vi "P4CMDSub Get Changelist Info.vi"(6 "operation message":string, 8 "error in (no error)":errorcluster, 9 "files":path[](array[path]), 10 "changelist":string, 11 "source control reference in":T1) -> (0 "error out":errorcluster, 1 "description":string, 2 "status":string, 3 "source control reference out":T1, 4 "changelist files array":string[](array[string]), 5 "date":string)   [LabVIEW 2020, in "NI_SCC_P4CMD.lvlib"]
uses:
  <vilib>/SourceControl/Providers/P4CMD/NI_SCC_P4CMD.lvlib
  <vilib>/SourceControl/sccapi/SCCAPI Refnum.ctl
  <vilib>/SourceControl/Providers/P4CMD/P4CMD Operations.ctl
  <vilib>/SourceControl/sccapi/NI_SCC.lvlib
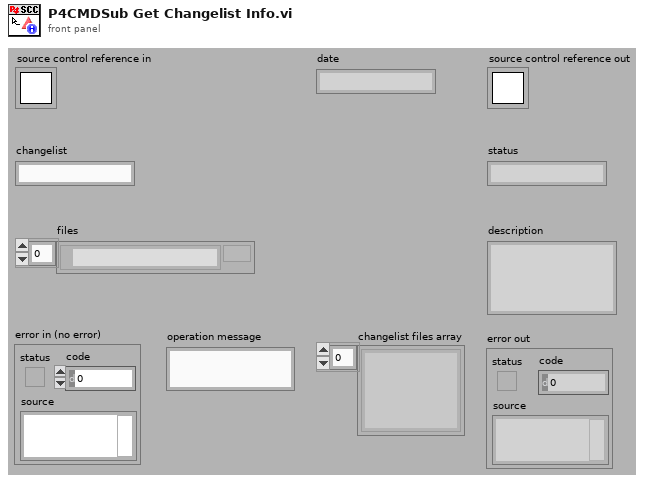
[diagram p1: front panel]
types:
  T1 = typedef "NI_SCC.lvlib/SCCAPI Refnum.ctl" = refnum<k1>
  T2 = typedef "NI_SCC_P4CMD.lvlib/P4CMD Operations.ctl" = enum16{"get all clients", "get all users", "describe changelist", "sync from depot", "open for edit", "submit to depot", "revert", "add to depot", "remove from depot", "print files revisions", "compare client file", "print depot file contents", "list opened files", "get file info", "lock files", "edit changelist spec", "info", "set variables"}
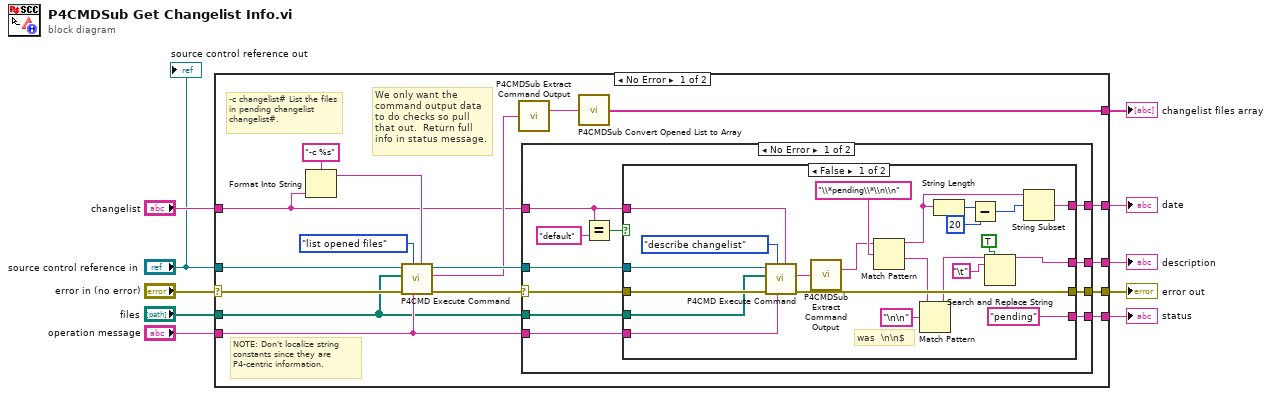
[diagram p0: block diagram]
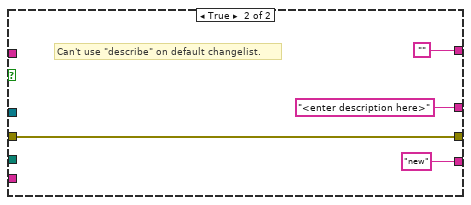
[diagram p2: hidden frame]
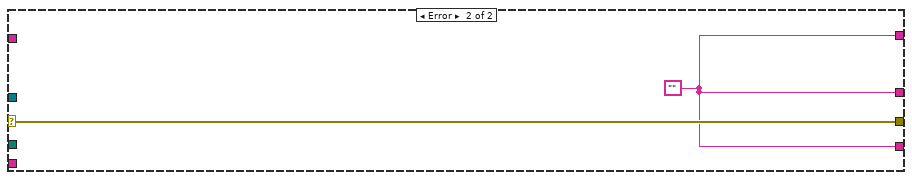
[diagram p4: hidden frame]
diagram:
  n1 = case shown="No Error" "error in (no error)" {
    selector: "error in (no error)" -> [w20 w67]
    tunnel: "changelist" -> [w11 _]
    tunnel: [w27 w66] -> w9
    tunnel: [w26 w66] -> w8
    tunnel: [w25 w67] -> w7
    tunnel: [w24 w66] -> w5
    tunnel: "files" -> [w16 _]
    tunnel: "source control reference in" -> [w22 _]
    tunnel: "operation message" -> [w18 _]
    tunnel: [w17 _] -> w2
    frame No Error {
      # "-c changelist# List the files in pending changelist changelist#."
      # "We only want the command output data to do checks so pull that out.  Return full info in status message."
      # "NOTE: Don't localize string constants since they are P4-centric information."
      n2 = Format Into String(format string="-c %s", w11) -> (resulting string=w12:string)  [unwired: 2 in, 1 out]
      n3 = call <vilib>:"P4CMD Execute Command.vi"("optional operation parameters"=w12, "operation message"=w18, "p4 operation"=P4CMD_Operations."list opened files", "error in (no error)"=w20, "files"=w16, "source control reference in"=w22) -> ("error out"=w19:errorcluster, "command information"=w15:string, "source control reference out"=w21:T1)  [unwired: 3 in]
      n4 = call <vilib>:"P4CMDSub Extract Command Output.vi"("bundled message"=w15) -> ("command output"=w14:string)  [unwired: 13 in, 1 out]
      n5 = case shown="No Error" w19 {
        selector: w19 -> [w28 w65]
        tunnel: w11 -> [w36 _]
        tunnel: [w35 _] -> w27
        tunnel: [w34 _] -> w26
        tunnel: [w33 w65] -> w25
        tunnel: [w32 _] -> w24
        tunnel: w16 -> [w31 _]
        tunnel: w18 -> [w30 _]
        tunnel: w21 -> [w29 _]
        frame No Error {
          n6 = Equal?(x=w36, y="default") -> (x = y?=w37:bool)
          n7 = case shown="False" w37 {
            tunnel: w36 -> [w42 _]
            tunnel: [w57 ""] -> w35
            tunnel: ["pending" ("command output") "new" ("command output")] -> w34
            tunnel: w28 -> [w59 w62]
            tunnel: [w58 w62] -> w33
            tunnel: [w50 "<enter description here>" ("command output")] -> w32
            tunnel: w31 -> [w41 _]
            tunnel: w30 -> [w46 _]
            tunnel: w29 -> [w43 _]
            frame False {
              # "was  \\n\\n$"
              n8 = call <vilib>:"P4CMD Execute Command.vi"("optional operation parameters"=w42, "operation message"=w46, "p4 operation"=P4CMD_Operations."describe changelist", "error in (no error)"=w59, "files"=w41, "source control reference in"=w43) -> ("error out"=w58:errorcluster, "command information"=w40:string)  [unwired: 3 in, 1 out]
              n9 = call <vilib>:"P4CMDSub Extract Command Output.vi"("bundled message"=w40) -> ("command output"=w39:string)  [unwired: 13 in, 1 out]
              n10 = Match Pattern(string=w39, regular expression="\\*pending\\*\\n\\n") -> (before substring=w52:string, after substring=w47:string)  [unwired: 1 in, 2 out]
              n11 = Match Pattern(string=w47, regular expression="\n\n") -> (before substring=w48:string)  [unwired: 1 in, 3 out]
              n12 = String Length(string=w52) -> (length=w55:i32)
              n13 = Subtract(x=w55, y=20) -> (x-y=w53:i32)
              n14 = Search and Replace String(replace all?=TRUE ("replace all? (F)"), input string=w48, search string="\t") -> (result string=w50:string)  [unwired: 5 in, 3 out]
              n15 = String Subset(string=w52, offset (0)=w53) -> (substring=w57:string)  [unwired: 1 in]
            }
            frame True {
              # "Can't use \"describe\" on default changelist."
            }
          }
        }
        frame Error {
        }
      }
      n16 = call <vilib>:"P4CMDSub Convert Opened List to Array.vi"("opened string"=w14) -> ("changelist files array"=w17:string[])  [unwired: 4 in]
    }
    frame Error {
      w66 = ""
    }
  }
  "date" <- w9
  "status" <- w8
  "error out" <- w7
  "description" <- w5
  "changelist files array" <- w2
  "source control reference out" <- "source control reference in"
